vi "test15-MappingRelationshipByLocalRegistration_State.vi"(8 "error in (no error)":errorcluster, 11 "TestCase in":refnum<class "testcase-CSMBroadcast.lvclass">) -> (0 "error out":errorcluster, 3 "TestCase out":refnum<class "testcase-CSMBroadcast.lvclass">)   [LabVIEW 2017, in "testcase-CSMBroadcast.lvclass"]
uses:
  testcase-CSMBroadcast.lvclass
  <vilib>/addons/_JKI Toolkits/VI Tester/TestCase.llb/TestCase.lvclass
  src/user.lib/_NEVSTOP/Communicable State Machine(CSM)/Communicable State Machine.lvlib
  C:/Program Files (x86)/National Instruments/LabVIEW 2017/vi.lib/addons/_JKI Toolkits/VI Tester/TestCase.llb/TestCase.lvclass
panel:
  out "Error Array 2":errorcluster[](array[cluster])
  out "Rules 3":T1(array[cluster])
  out "Status In Registry 3":string[](array[string])
  out "Rules 4":T1(array[cluster])
  out "Status In Registry 4":string[](array[string])
  out "Loop Count 2":i32
  out "Loop Count":i32
  out "Error Array":errorcluster[](array[cluster])
  out "Rules 2":T1(array[cluster])
  out "Status In Registry 2":string[](array[string])
  out "Status In Registry 1":string[](array[string])
  out "Rules 1":T1(array[cluster])
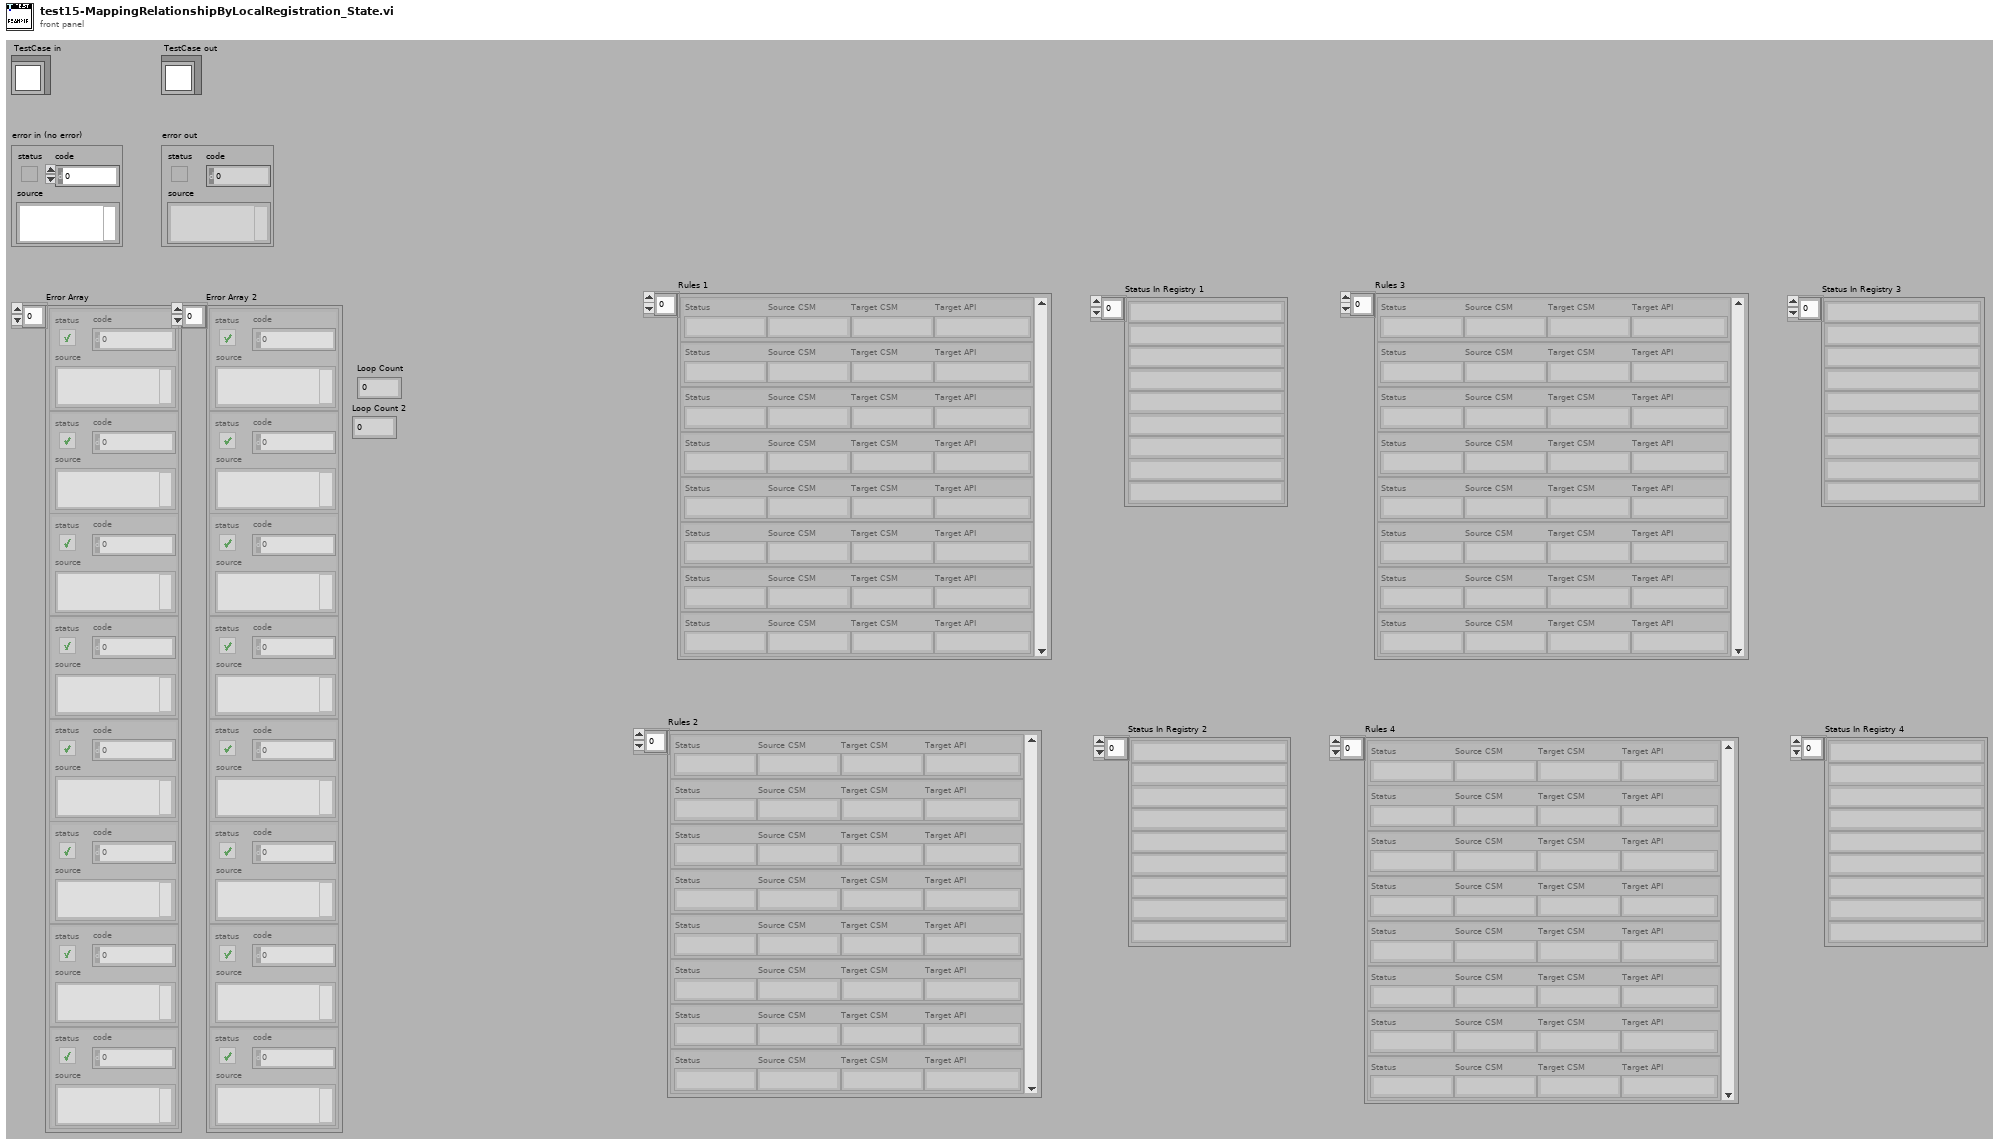
[diagram p1: front panel]
types:
  T1 = cluster{"Status":string, "Source CSM":string, "Target CSM":string, "Target API":string}[]
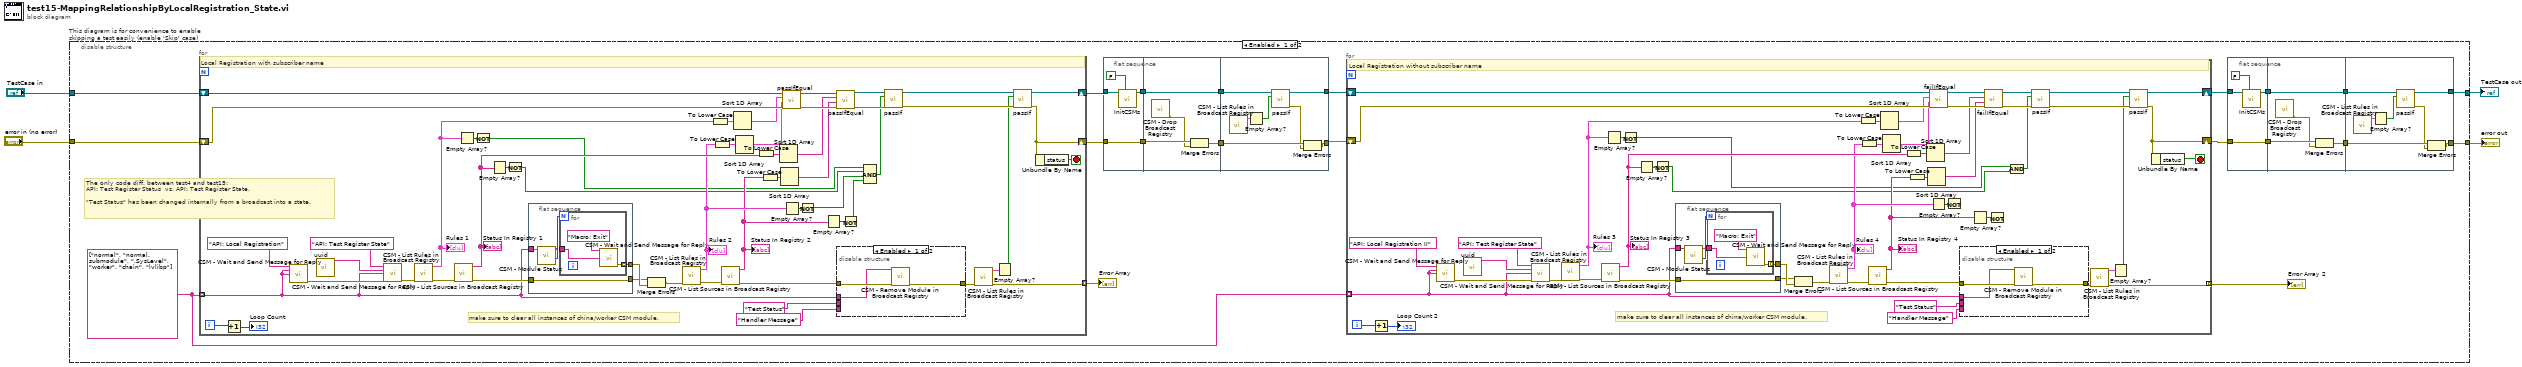
[diagram p0: block diagram]
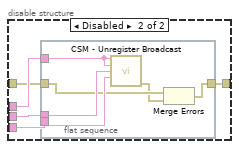
[diagram p2: hidden frame]
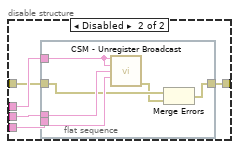
[diagram p3: hidden frame]
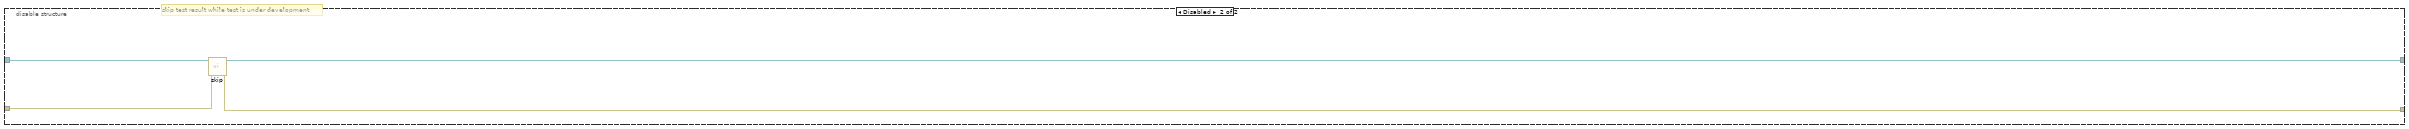
[diagram p4: hidden frame]
diagram:
  n1 = disable-structure "This diagram is for convenience to enable skipping a test easily (enable 'Skip' case)" shown="Enabled" {
    disable-tunnel: "TestCase in" -> [w25 w207]
    disable-tunnel: [w7 w205] -> w1
    disable-tunnel: [w5 w206] -> w3
    disable-tunnel: "error in (no error)" -> [w21 w204]
    frame Enabled {
      w22 = string[] ["normal", "normal.submodule", ".SysLevel", "worker", "chain", "lvlibp"]
      # "The only code diff. between test4 and test15:\nAPI: Test Register Status  vs. API: Test Register State.\n\n\"Test Status\" has been changed internally from a broadcast into a state."
      n2 = for {
        tunnel: w22 -> [w139] mode=indexing
        shift-right: [w130] -> w18
        shift-left: w25 -> [w174]
        shift-right: [w132] -> w17
        shift-left: w21 -> [w173]
        tunnel: [w135] -> w24 mode=indexing
        i -> [w159]
        stop <- w172 stop-if-true
        # "make sure to clear all instances of china/worker CSM module."
        # "Local Registration with subscriber name"
        n3 = Increment(x=w159) -> (x+1=→"Loop Count":i32)
        n4 = call "CSM - Wait and Send Message for Reply.vi"("State"="API: Local Registration", "Arguments (\"\")"=w139, "Target Module"=w139) -> ("error out"=w180:errorcluster)  [unwired: 9 in, 3 out]
        n5 = call "uuid.vi"() -> ("UUID"=w178:string)  [unwired: 11 in]
        n6 = call "CSM - Wait and Send Message for Reply.vi"("State"="API: Test Register State", "Arguments (\"\")"=w178, "Target Module"=w139, "Error In (No Error)"=w180) -> ("error out"=w177:errorcluster)  [unwired: 8 in, 3 out]
        n7 = call "CSM - List Rules in Broadcast Registry.vi"("error in (no error)"=w177) -> ("error out"=w171:errorcluster, "Rule Entries"=w155:T1)  [unwired: 8 in, 1 out]
        "Rules 1" <- w155
        n8 = call "CSM - List Sources in Broadcast Registry.vi"("error in (no error)"=w171) -> ("error out"=w157:errorcluster, "Broadcast Names"=w152:string[])  [unwired: 9 in]
        "Status In Registry 1" <- w152
        n9 = Empty Array?(array=w155) -> (empty?=w154:bool)
        n10 = Not(x=w154) -> (.not. x?=w147:bool)
        n11 = Empty Array?(array=w152) -> (empty?=w153:bool)
        n12 = Not(x=w153) -> (.not. x?=w146:bool)
        n13 = flat-sequence {
          tunnel: [w200] -> w176
          tunnel: w139 -> [w198]
          tunnel: [w197] -> w156
          tunnel: w157 -> [w197]
          frame #0 {
            n14 = call "CSM - Module Status.vi"("CSM Name"=w198) -> ("#Nodes"=w199:i32, "CSM Name (Dup)"=w196:string)  [unwired: 6 in, 3 out]
            n15 = for {
              N: w199 -> [_]
              tunnel: [w202] -> w200 mode=indexing
              tunnel: w196 -> [w201]
              n16 = call "CSM - Wait and Send Message for Reply.vi"("State"="Macro: Exit", "Target Module"=w201) -> ("error out"=w202:errorcluster)  [unwired: 10 in, 3 out]
            }
          }
        }
        n17 = Merge Errors(w156, w176) -> (w175:errorcluster)
        n18 = call "CSM - List Rules in Broadcast Registry.vi"("error in (no error)"=w175) -> ("error out"=w170:errorcluster, "Rule Entries"=w150:T1)  [unwired: 8 in, 1 out]
        "Rules 2" <- w150
        n19 = To Lower Case(string=w155) -> (all lower case string=w169:T1)
        n20 = To Lower Case(string=w150) -> (all lower case string=w168:T1)
        n21 = call "CSM - List Sources in Broadcast Registry.vi"("error in (no error)"=w170) -> ("error out"=w140:errorcluster, "Broadcast Names"=w148:string[])  [unwired: 9 in]
        "Status In Registry 2" <- w148
        n22 = Sort 1D Array(array=w169) -> (sorted array=w167:T1)
        n23 = Sort 1D Array(array=w168) -> (sorted array=w166:T1)
        n24 = To Lower Case(string=w152) -> (all lower case string=w163:string[])
        n25 = To Lower Case(string=w148) -> (all lower case string=w162:string[])
        n26 = Sort 1D Array(array=w163) -> (sorted array=w161:string[])
        n27 = Sort 1D Array(array=w162) -> (sorted array=w160:string[])
        n28 = call-dynamic "passIfEqual.vi"("error in (no error)"=w173, "y"=w166, "x"=w167, "TestCase in"=w174) -> ("error out"=w164:errorcluster, "TestCase out"=w165:refnum<class "testcase-CSMBroadcast.lvclass">)  [unwired: 6 in]
        n29 = Empty Array?(array=w150) -> (empty?=w151:bool)
        n30 = Not(x=w151) -> (.not. x?=w145:bool)
        n31 = Empty Array?(array=w148) -> (empty?=w149:bool)
        n32 = disable-structure shown="Enabled" {
          disable-tunnel: w140 -> [w184 w186]
          disable-tunnel: [w183 w185] -> w136
          disable-tunnel: w139 -> [w182 w187]
          disable-tunnel: "Test Status" ("Status") -> [_ w189]
          disable-tunnel: "Handler Message" ("Response Message (If \"\", Same as Source Message)") -> [_ w188]
          frame Enabled {
            n33 = call "CSM - Remove Module in Broadcast Registry.vi"("CSM Name"=w182, "Error In"=w184) -> ("error out"=w183:errorcluster)  [unwired: 12 in, 1 out]
          }
          frame Disabled {
            n34 = flat-sequence {
              tunnel: w189 -> [w195]
              tunnel: w188 -> [w194]
              tunnel: w187 -> [w193]
              tunnel: w186 -> [w192]
              tunnel: [w190] -> w185
              frame #0 {
                n35 = call "CSM - Unregister Broadcast.vi"("CSM Name(Empty for Broadcast Event)"=w193, "Source CSM Name (* as Default)"=w193, "Trigger"=w195, "API (\"*\" as Default)"=w194) -> ("error out"=w191:errorcluster)  [unwired: 10 in, 1 out]
                n36 = Merge Errors(w192, w191) -> (w190:errorcluster)
              }
            }
          }
        }
        n37 = call-dynamic "passIfEqual.vi"("error in (no error)"=w164, "y"=w160, "x"=w161, "TestCase in"=w165) -> ("error out"=w142:errorcluster, "TestCase out"=w143:refnum<class "testcase-CSMBroadcast.lvclass">)  [unwired: 6 in]
        n38 = Not(x=w149) -> (.not. x?=w144:bool)
        n39 = Compound Arithmetic op=AND(w147, w146, w145, w144) -> (w141:bool)
        n40 = call-dynamic "passIf.vi"("error in (no error)"=w142, "pass"=w141, "TestCase in"=w143) -> ("error out"=w133:errorcluster, "TestCase out"=w131:refnum<class "testcase-CSMBroadcast.lvclass">)  [unwired: 7 in]
        n41 = call "CSM - List Rules in Broadcast Registry.vi"("error in (no error)"=w136) -> ("error out"=w135:errorcluster, "Rule Entries"=w134:T1)  [unwired: 8 in, 1 out]
        n42 = Empty Array?(array=w134) -> (empty?=w129:bool)
        n43 = call-dynamic "passIf.vi"("error in (no error)"=w133, "pass"=w129, "TestCase in"=w131) -> ("error out"=w132:errorcluster, "TestCase out"=w130:refnum<class "testcase-CSMBroadcast.lvclass">)  [unwired: 7 in]
        n44 = Unbundle By Name(w132) -> ("status"=w172:bool)
      }
      "Error Array" <- w24
      n45 = flat-sequence {
        tunnel: w18 -> [w44]
        tunnel: [w43] -> w20
        tunnel: [w42] -> w19
        tunnel: w17 -> [w42]
        tunnel: w20 -> [w48]
        tunnel: w19 -> [w47]
        tunnel: [w48] -> w14
        tunnel: [w46] -> w13
        tunnel: [w50] -> w15
        tunnel: [w53] -> w16
        tunnel: w14 -> [w54]
        tunnel: w13 -> [w55]
        frame #0 {
          n46 = call "InitCSMs.vi"("Enable building lvlibp?"=FALSE, "testcase-CSMStatus in"=w44) -> ("testcase-CSMStatus out"=w43:refnum<class "testcase-CSMBroadcast.lvclass">)  [unwired: 8 in, 1 out]
        }
        frame #1 {
          n47 = call "CSM - Drop Broadcast Registry.vi"() -> ("error out"=w45:errorcluster)  [unwired: 15 in]
          n48 = Merge Errors(w47, w45) -> (w46:errorcluster)
        }
        frame #2 {
          n49 = call "CSM - List Rules in Broadcast Registry.vi"() -> ("Rule Entries"=w52:T1)  [unwired: 9 in, 2 out]
          n50 = Empty Array?(array=w52) -> (empty?=w51:bool)
          n51 = call-dynamic "passIf.vi"("pass"=w51, "TestCase in"=w54) -> ("error out"=w49:errorcluster, "TestCase out"=w53:refnum<class "testcase-CSMBroadcast.lvclass">)  [unwired: 8 in]
          n52 = Merge Errors(w55, w49) -> (w50:errorcluster)
        }
      }
      n53 = for {
        tunnel: w22 -> [w66] mode=indexing
        shift-right: [w59] -> w8
        shift-left: w16 -> [w99]
        shift-right: [w57] -> w6
        shift-left: w15 -> [w98]
        tunnel: [w61] -> w23 mode=indexing
        i -> [w84]
        stop <- w97 stop-if-true
        # "make sure to clear all instances of china/worker CSM module."
        # "Local Registration without subscriber name"
        n54 = Increment(x=w84) -> (x+1=→"Loop Count 2":i32)
        n55 = call "CSM - Wait and Send Message for Reply.vi"("State"="API: Local Registration II", "Arguments (\"\")"=w66, "Target Module"=w66) -> ("error out"=w105:errorcluster)  [unwired: 9 in, 3 out]
        n56 = call "uuid.vi"() -> ("UUID"=w103:string)  [unwired: 11 in]
        n57 = call "CSM - Wait and Send Message for Reply.vi"("State"="API: Test Register State", "Arguments (\"\")"=w103, "Target Module"=w66, "Error In (No Error)"=w105) -> ("error out"=w102:errorcluster)  [unwired: 8 in, 3 out]
        n58 = call "CSM - List Rules in Broadcast Registry.vi"("error in (no error)"=w102) -> ("error out"=w96:errorcluster, "Rule Entries"=w80:T1)  [unwired: 8 in, 1 out]
        "Rules 3" <- w80
        n59 = call "CSM - List Sources in Broadcast Registry.vi"("error in (no error)"=w96) -> ("error out"=w82:errorcluster, "Broadcast Names"=w77:string[])  [unwired: 9 in]
        "Status In Registry 3" <- w77
        n60 = Empty Array?(array=w80) -> (empty?=w79:bool)
        n61 = Not(x=w79) -> (.not. x?=w72:bool)
        n62 = Empty Array?(array=w77) -> (empty?=w78:bool)
        n63 = Not(x=w78) -> (.not. x?=w71:bool)
        n64 = flat-sequence {
          tunnel: [w125] -> w101
          tunnel: w66 -> [w123]
          tunnel: [w122] -> w81
          tunnel: w82 -> [w122]
          frame #0 {
            n65 = call "CSM - Module Status.vi"("CSM Name"=w123) -> ("#Nodes"=w124:i32, "CSM Name (Dup)"=w121:string)  [unwired: 6 in, 3 out]
            n66 = for {
              N: w124 -> [_]
              tunnel: [w127] -> w125 mode=indexing
              tunnel: w121 -> [w126]
              n67 = call "CSM - Wait and Send Message for Reply.vi"("State"="Macro: Exit", "Target Module"=w126) -> ("error out"=w127:errorcluster)  [unwired: 10 in, 3 out]
            }
          }
        }
        n68 = Merge Errors(w81, w101) -> (w100:errorcluster)
        n69 = call "CSM - List Rules in Broadcast Registry.vi"("error in (no error)"=w100) -> ("error out"=w95:errorcluster, "Rule Entries"=w75:T1)  [unwired: 8 in, 1 out]
        "Rules 4" <- w75
        n70 = To Lower Case(string=w80) -> (all lower case string=w94:T1)
        n71 = To Lower Case(string=w75) -> (all lower case string=w93:T1)
        n72 = call "CSM - List Sources in Broadcast Registry.vi"("error in (no error)"=w95) -> ("error out"=w67:errorcluster, "Broadcast Names"=w73:string[])  [unwired: 9 in]
        "Status In Registry 4" <- w73
        n73 = Sort 1D Array(array=w94) -> (sorted array=w92:T1)
        n74 = Sort 1D Array(array=w93) -> (sorted array=w91:T1)
        n75 = To Lower Case(string=w77) -> (all lower case string=w88:string[])
        n76 = To Lower Case(string=w73) -> (all lower case string=w87:string[])
        n77 = Sort 1D Array(array=w88) -> (sorted array=w86:string[])
        n78 = Sort 1D Array(array=w87) -> (sorted array=w85:string[])
        n79 = call-dynamic "failIfEqual.vi"("error in (no error)"=w98, "y"=w91, "x"=w92, "TestCase in"=w99) -> ("error out"=w89:errorcluster, "TestCase out"=w90:refnum<class "testcase-CSMBroadcast.lvclass">)  [unwired: 6 in]
        n80 = Empty Array?(array=w75) -> (empty?=w76:bool)
        n81 = Not(x=w76) -> ()  [unwired: 1 out]
        n82 = disable-structure shown="Enabled" {
          disable-tunnel: w67 -> [w109 w111]
          disable-tunnel: [w108 w110] -> w62
          disable-tunnel: w66 -> [w107 w112]
          disable-tunnel: "Test Status" ("Status") -> [_ w114]
          disable-tunnel: "Handler Message" ("Response Message (If \"\", Same as Source Message)") -> [_ w113]
          frame Enabled {
            n83 = call "CSM - Remove Module in Broadcast Registry.vi"("CSM Name"=w107, "Error In"=w109) -> ("error out"=w108:errorcluster)  [unwired: 12 in, 1 out]
          }
          frame Disabled {
            n84 = flat-sequence {
              tunnel: w114 -> [w120]
              tunnel: w113 -> [w119]
              tunnel: w112 -> [w118]
              tunnel: w111 -> [w117]
              tunnel: [w115] -> w110
              frame #0 {
                n85 = call "CSM - Unregister Broadcast.vi"("CSM Name(Empty for Broadcast Event)"=w118, "Source CSM Name (* as Default)"=w118, "Trigger"=w120, "API (\"*\" as Default)"=w119) -> ("error out"=w116:errorcluster)  [unwired: 10 in, 1 out]
                n86 = Merge Errors(w117, w116) -> (w115:errorcluster)
              }
            }
          }
        }
        n87 = Empty Array?(array=w73) -> (empty?=w74:bool)
        n88 = call-dynamic "failIfEqual.vi"("error in (no error)"=w89, "y"=w85, "x"=w86, "TestCase in"=w90) -> ("error out"=w69:errorcluster, "TestCase out"=w70:refnum<class "testcase-CSMBroadcast.lvclass">)  [unwired: 6 in]
        n89 = Not(x=w74) -> ()  [unwired: 1 out]
        n90 = Compound Arithmetic op=AND(w72, w71) -> (w68:bool)
        n91 = call-dynamic "passIf.vi"("error in (no error)"=w69, "pass"=w68, "TestCase in"=w70) -> ("error out"=w58:errorcluster, "TestCase out"=w60:refnum<class "testcase-CSMBroadcast.lvclass">)  [unwired: 7 in]
        n92 = call "CSM - List Rules in Broadcast Registry.vi"("error in (no error)"=w62) -> ("error out"=w61:errorcluster, "Rule Entries"=w63:T1)  [unwired: 8 in, 1 out]
        n93 = Empty Array?(array=w63) -> (empty?=w56:bool)
        n94 = call-dynamic "passIf.vi"("error in (no error)"=w58, "pass"=w56, "TestCase in"=w60) -> ("error out"=w57:errorcluster, "TestCase out"=w59:refnum<class "testcase-CSMBroadcast.lvclass">)  [unwired: 7 in]
        n95 = Unbundle By Name(w57) -> ("status"=w97:bool)
      }
      "Error Array 2" <- w23
      n96 = flat-sequence {
        tunnel: w8 -> [w29]
        tunnel: [w28] -> w12
        tunnel: [w27] -> w11
        tunnel: w6 -> [w27]
        tunnel: w12 -> [w33]
        tunnel: w11 -> [w32]
        tunnel: [w33] -> w10
        tunnel: [w31] -> w9
        tunnel: [w35] -> w5
        tunnel: [w38] -> w7
        tunnel: w10 -> [w39]
        tunnel: w9 -> [w40]
        frame #0 {
          n97 = call "InitCSMs.vi"("Enable building lvlibp?"=FALSE, "testcase-CSMStatus in"=w29) -> ("testcase-CSMStatus out"=w28:refnum<class "testcase-CSMBroadcast.lvclass">)  [unwired: 8 in, 1 out]
        }
        frame #1 {
          n98 = call "CSM - Drop Broadcast Registry.vi"() -> ("error out"=w30:errorcluster)  [unwired: 15 in]
          n99 = Merge Errors(w32, w30) -> (w31:errorcluster)
        }
        frame #2 {
          n100 = call "CSM - List Rules in Broadcast Registry.vi"() -> ("Rule Entries"=w37:T1)  [unwired: 9 in, 2 out]
          n101 = Empty Array?(array=w37) -> (empty?=w36:bool)
          n102 = call-dynamic "passIf.vi"("pass"=w36, "TestCase in"=w39) -> ("error out"=w34:errorcluster, "TestCase out"=w38:refnum<class "testcase-CSMBroadcast.lvclass">)  [unwired: 8 in]
          n103 = Merge Errors(w40, w34) -> (w35:errorcluster)
        }
      }
    }
    frame Disabled {
      # "skip test result while test is under development"
      n104 = call <vilib>:"skip.vi"("error in (no error)"=w204, "TestCase in"=w207) -> ("error out"=w206:errorcluster, "TestCase out"=w205:refnum<class "testcase-CSMBroadcast.lvclass">)  [unwired: 8 in]
    }
  }
  "error out" <- w3
  "TestCase out" <- w1
